vi "Filter - level range.vi"(8 "error in (no error)":errorcluster) -> (0 "error out":errorcluster)   [LabVIEW 2026, in "Tests.lvlib"]
doc: "Unit test (Caraya). Verifies RoutedFilterMatch level-band behavior and the level-AND-tag conjunction: a single-level band accepts only that level, a level more severe than levelMin or less severe than levelMax is rejected, an in-band level is accepted, and an in-band level with a non-matching tag is still rejected (SRS-LMBR-026). Tag is held matching except the final conjunction case. Pure, no fixtures.\n\nImplements LMBR-T-014 -> SRS-026, SRS-027; LMBR-T-015 -> SRS-026. Assert-level IDs: Test-ID-Assert-Checklist.md."
uses:
  Tests.lvlib
  src/TypeDefs/Statement.ctl
  src/TypeDefs/Severity.ctl
  src/TypeDefs/Filter.ctl
  src/TypeDefs/FilterMode.ctl
  <vilib>/addons/_JKI Toolkits/Caraya/classes/Assert/Assert True.vi
  <vilib>/addons/_JKI Toolkits/Caraya/classes/Assert/Assert False.vi
  <vilib>/addons/_JKI Toolkits/Caraya/classes/Test/Test.lvclass
  <vilib>/addons/_JKI Toolkits/Caraya/classes/Assert/Assert.lvclass
  src/Lumberjack.lvlib
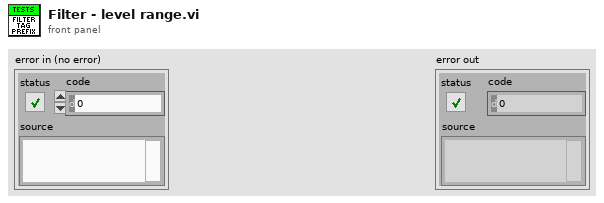
[diagram p1: front panel]
types:
  T1 = typedef "Lumberjack.lvlib/Severity.ctl" = enum16{"OFF", "FATAL", "ERROR", "WARN", "INFO", "DEBUG", "TRACE", "ALL"}
  T2 = typedef "Lumberjack.lvlib/Filter.ctl" = cluster{"mode":T3, "levelMin":T1, "levelMax":T1, "tagPrefix":string}
  T3 = typedef "Lumberjack.lvlib/FilterMode.ctl" = enum16{"Mirror", "Routed"}
  T4 = typedef "Lumberjack.lvlib/Statement.ctl" = cluster{"timestamp":timestamp, "level":T1, "sourceTag":string, "originVI":string, "message":string}
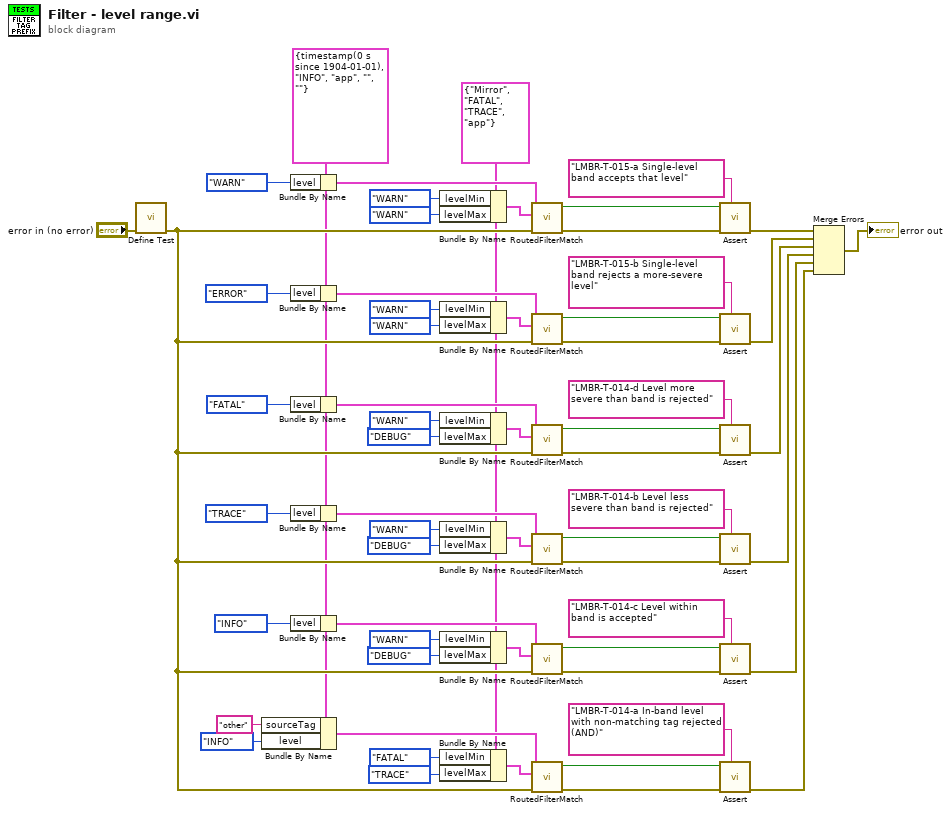
[diagram p0: block diagram]
diagram:
  w14 = T2 {"mode"=enum."Mirror", "levelMin"=enum."FATAL", "levelMax"=enum."TRACE", "tagPrefix"="app"} ("Filter")
  w15 = T4 {"timestamp"=timestamp(0 s since 1904-01-01), "level"=enum."INFO", "sourceTag"="app", "originVI"="", "message"=""} ("Statement")
  n1 = call <vilib>:"Define Test.vi"("error in (no error)"="error in (no error)") -> ("error out"=w17:errorcluster)  [unwired: 9 in, 1 out]
  n2 = Bundle By Name(cluster=w15, "sourceTag"="other", "level"=Severity."INFO") -> (w22:T4)
  n3 = Bundle By Name(cluster=w15, "level"=Severity."WARN") -> (w56:T4)
  n4 = Bundle By Name(cluster=w15, "level"=Severity."ERROR") -> (w51:T4)
  n5 = Bundle By Name(cluster=w15, "level"=Severity."FATAL") -> (w46:T4)
  n6 = Bundle By Name(cluster=w15, "level"=Severity."TRACE") -> (w41:T4)
  n7 = Bundle By Name(cluster=w15, "level"=Severity."INFO") -> (w36:T4)
  n8 = Bundle By Name(cluster=w14, "levelMin"=Severity."WARN", "levelMax"=Severity."WARN") -> (w53:T2)
  n9 = Bundle By Name(cluster=w14, "levelMin"=Severity."WARN", "levelMax"=Severity."WARN") -> (w48:T2)
  n10 = Bundle By Name(cluster=w14, "levelMin"=Severity."WARN", "levelMax"=Severity."DEBUG") -> (w43:T2)
  n11 = Bundle By Name(cluster=w14, "levelMin"=Severity."WARN", "levelMax"=Severity."DEBUG") -> (w38:T2)
  n12 = Bundle By Name(cluster=w14, "levelMin"=Severity."WARN", "levelMax"=Severity."DEBUG") -> (w33:T2)
  n13 = Bundle By Name(cluster=w14, "levelMin"=Severity."FATAL", "levelMax"=Severity."TRACE") -> (w19:T2)
  n14 = call "RoutedFilterMatch.vi"("error in (no error)"=w17, "Filter"=w53, "Statement"=w56) -> ("error out"=w57:errorcluster, "Accepted"=w54:bool)  [unwired: 7 in]
  n15 = call "RoutedFilterMatch.vi"("error in (no error)"=w17, "Filter"=w48, "Statement"=w51) -> ("error out"=w52:errorcluster, "Accepted"=w49:bool)  [unwired: 7 in]
  n16 = call "RoutedFilterMatch.vi"("error in (no error)"=w17, "Filter"=w43, "Statement"=w46) -> ("error out"=w47:errorcluster, "Accepted"=w44:bool)  [unwired: 7 in]
  n17 = call "RoutedFilterMatch.vi"("error in (no error)"=w17, "Filter"=w38, "Statement"=w41) -> ("error out"=w42:errorcluster, "Accepted"=w39:bool)  [unwired: 7 in]
  n18 = call "RoutedFilterMatch.vi"("error in (no error)"=w17, "Filter"=w33, "Statement"=w36) -> ("error out"=w37:errorcluster, "Accepted"=w34:bool)  [unwired: 7 in]
  n19 = call "RoutedFilterMatch.vi"("error in (no error)"=w17, "Filter"=w19, "Statement"=w22) -> ("error out"=w23:errorcluster, "Accepted"=w20:bool)  [unwired: 7 in]
  n20 = call-poly <vilib>:"Assert.vi"("Label"="LMBR-T-015-a Single-level band accepts that level", "error in (no error)"=w57, "True?"=w54) -> ("error out"=w58:errorcluster)  [unwired: 7 in, 1 out]
  n21 = call-poly <vilib>:"Assert.vi"("Label"="LMBR-T-015-b Single-level band rejects a more-severe level", "error in (no error)"=w52, "False?"=w49) -> ("error out"=w32:errorcluster)  [unwired: 7 in, 1 out]
  n22 = call-poly <vilib>:"Assert.vi"("Label"="LMBR-T-014-d Level more severe than band is rejected", "error in (no error)"=w47, "False?"=w44) -> ("error out"=w31:errorcluster)  [unwired: 7 in, 1 out]
  n23 = call-poly <vilib>:"Assert.vi"("Label"="LMBR-T-014-b Level less severe than band is rejected", "error in (no error)"=w42, "False?"=w39) -> ("error out"=w30:errorcluster)  [unwired: 7 in, 1 out]
  n24 = call-poly <vilib>:"Assert.vi"("Label"="LMBR-T-014-c Level within band is accepted", "error in (no error)"=w37, "True?"=w34) -> ("error out"=w29:errorcluster)  [unwired: 7 in, 1 out]
  n25 = call-poly <vilib>:"Assert.vi"("Label"="LMBR-T-014-a In-band level with non-matching tag rejected (AND)", "error in (no error)"=w23, "False?"=w20) -> ("error out"=w16:errorcluster)  [unwired: 7 in, 1 out]
  n26 = Merge Errors(w58, w32, w31, w30, w29, w16) -> (→"error out":errorcluster)
